vi "getReadTagBusRef.vi"(8 "error in (no error)":errorcluster) -> (0 "error out":errorcluster, 1 "valid references":bool, 2 "read data table":refnum<queue>, 3 "read data dictionary":refnum<queue>)   [LabVIEW 2013]
uses:
  <vilib>/NI/Tag Bus/dictionary/data dictionary.lvclass
  <vilib>/NI/Tag Bus/table/data table.ctl
  <vilib>/NI/Tag Bus/table/data table.lvlib
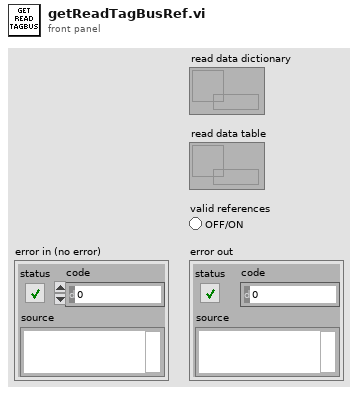
[diagram p1: front panel]
types:
  T1 = typedef "tag bus.lvlib/data table.lvlib/data table.ctl" = cluster{"Double":dbl[], "Single":sgl[], "I64":i64[], "I32":i32[], "I16":i16[], "I8":i8[], "U64":u64[], "U32":u32[], "U16":u16[], "U8":u8[], "Boolean":bool[], "String":string[], "Array of Double":cluster{"DBL Array":dbl[]}[], "Array of Single":cluster{"SGL Array":sgl[]}[], "Array of I64":cluster{"I64 Array":i64[]}[], "Array of I32":cluster{"I32 Array":i32[]}[], "Array of I16":cluster{"I16 Array":i16[]}[], "Array of I8":cluster{"I8 Array":i8[]}[], "Array of U64":cluster{"U64 Array":u64[]}[], "Array of U32":cluster{"U32 Array":u32[]}[], "Array of U16":cluster{"U16 Array":u16[]}[], "Array of U8":cluster{"U8 Array":u8[]}[], "Array of Boolean":cluster{"Boolean Array":bool[]}[], "Array of String":cluster{"String Array":string[]}[]}
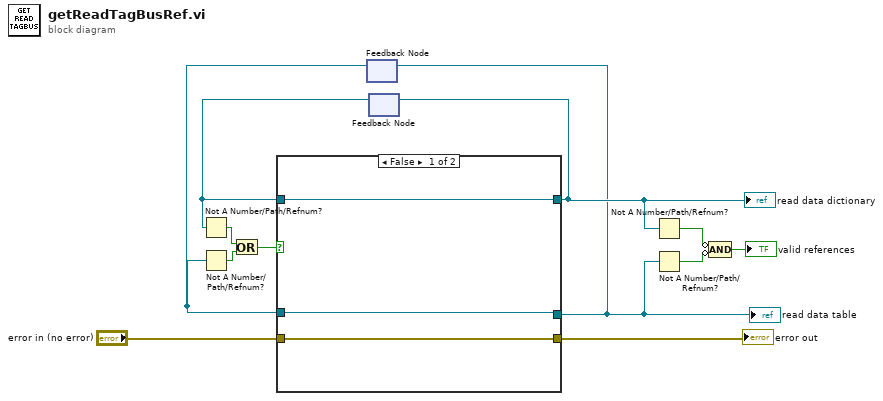
[diagram p0: block diagram]
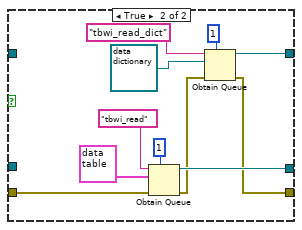
[diagram p2: hidden frame]
diagram:
  n1 = feedback #1() -> (w8:refnum<queue>)  [unwired: 1 in]
  n2 = Not A Number/Path/Refnum?(number/path/refnum=w8) -> (NaN/Path/Refnum?=w10:bool)
  n3 = feedback #2() -> (w12:refnum<queue>)  [unwired: 1 in]
  n4 = Not A Number/Path/Refnum?(number/path/refnum=w12) -> (NaN/Path/Refnum?=w9:bool)
  n5 = Or(x=w9, y=w10) -> (x .or. y?=w11:bool)
  n6 = case shown="False" w11 {
    tunnel: [w14 w18] -> w6
    tunnel: [w15 w24] -> w4
    tunnel: w8 -> [w15 _]
    tunnel: "error in (no error)" -> [w14 w23]
    tunnel: [w13 w20] -> w5
    tunnel: w12 -> [w13 _]
    frame False {
    }
    frame True {
      n7 = Obtain Queue(max queue size (-1, unlimited)=1, name (unnamed)="tbwi_read", element data type=T1 {"Double"=[], "Single"=[], "I64"=[], "I32"=[], "I16"=[], "I8"=[], "U64"=[], "U32"=[], "U16"=[], "U8"=[], "Boolean"=[], "String"=[], "Array of Double"=[], "Array of Single"=[], "Array of I64"=[], "Array of I32"=[], "Array of I16"=[], "Array of I8"=[], "Array of U64"=[], "Array of U32"=[], "Array of U16"=[], "Array of U8"=[], "Array of Boolean"=[], "Array of String"=[]} ("Data Interface out"), error in (no error)=w23) -> (queue out=w24:refnum<queue>, error out=w19:errorcluster)  [unwired: 1 in, 1 out]
      n8 = Obtain Queue(max queue size (-1, unlimited)=1, name (unnamed)="tbwi_read_dict", element data type=refnum<class "data dictionary.lvclass"> refnum ("input data.data dictionary"), error in (no error)=w19) -> (queue out=w20:refnum<queue>, error out=w18:errorcluster)  [unwired: 1 in, 1 out]
    }
  }
  "read data dictionary" <- w5
  "error out" <- w6
  "read data table" <- w4
  n9 = feedback-in #1(w4) -> ()
  n10 = feedback-in #2(w5) -> ()
  n11 = Not A Number/Path/Refnum?(number/path/refnum=w5) -> (NaN/Path/Refnum?=w3:bool)
  n12 = Not A Number/Path/Refnum?(number/path/refnum=w4) -> (NaN/Path/Refnum?=w2:bool)
  n13 = Compound Arithmetic op=AND(invert w3, invert w2) -> (→"valid references":bool)
